vi "LBCB Initialization & Autobalancing.vi"(0 "Selected LBCB":T1, 3 "error in (no error)":errorcluster) -> (8 "Use Previous\nCommand":bool, 10 "error out":errorcluster)   [LabVIEW 2009]
uses:
  lib/Data Access Objects/Metadata/LBCB Number.ctl
  lib/Global Data/Transactions/Dataset Transaction Id.ctl
  lib/Global Data/Transactions/Dataset Source.ctl
  lib/Global Data/Transactions/Dataset Type.ctl
  lib/Apps/Yes No Button.ctl
  lib/Data Access Objects/Metadata/DAO Actions.ctl
panel:
  in  "Autobalance":bool
  in  "Previous Command":bool
  out "Current Displacements":dbl[](array[numeric])
  in  "Previous Command Values":dbl[](array[numeric])
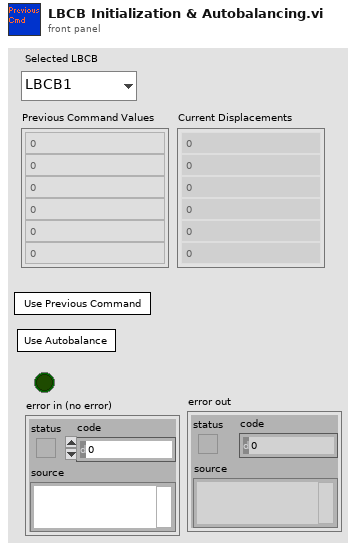
[diagram p1: front panel]
types:
  T1 = typedef "LBCB Number.ctl" = enum16{"LBCB1", "LBCB2"}
  T2 = typedef "Dataset Transaction Id.ctl" = cluster{"Dataset Source":T3, "Dataset Type":T4, "Hold":T5, "Volts":T5, "Tag":string}
  T3 = typedef "Dataset Source.ctl" = enum16{"LBCB 1", "LBCB 2", "Combined", "External Sensors"}
  T4 = typedef "Dataset Type.ctl" = enum16{"LVDT", "Load Cell", "Actuator Command", "Servo Error", "Displacement Command", "Displacement", "Force"}
  T5 = typedef "Yes No Button.ctl" = bool
  T6 = typedef "DAO Actions.ctl" = enum16{"Init", "Get", "Set"}
  T7 = typedef "Actuator Point.ctl" = cluster{"X1":dbl, "X2":dbl, "Y1":dbl, "Z1":dbl, "Z2":dbl, "Z3":dbl}
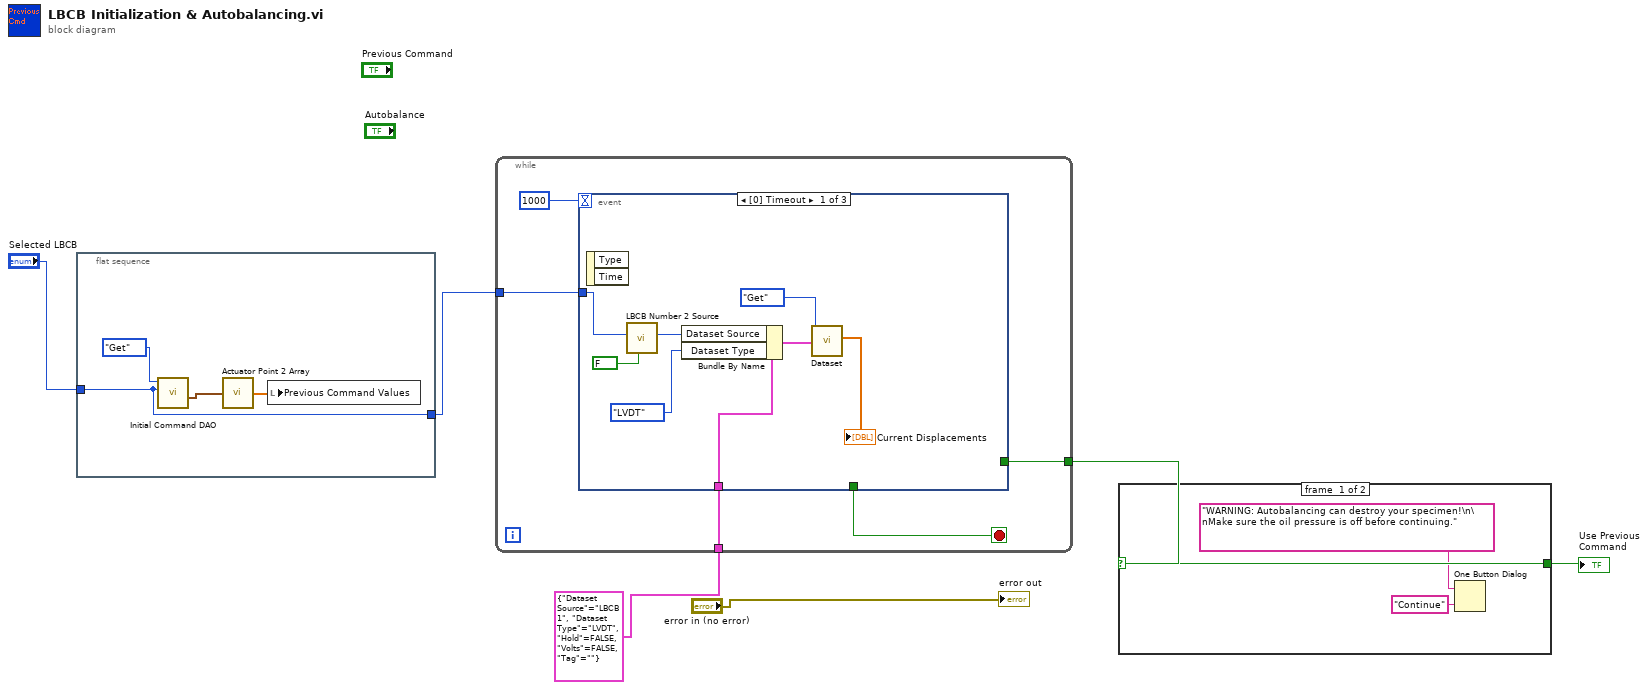
[diagram p0: block diagram]
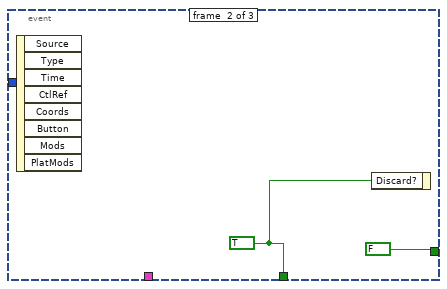
[diagram p3: hidden frame]
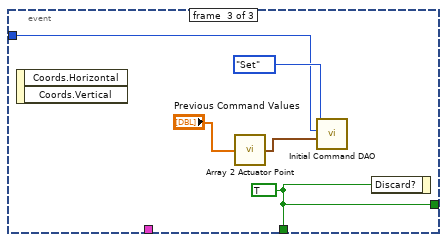
[diagram p4: hidden frame]
diagram:
  n1 = flat-sequence {
    tunnel: "Selected LBCB" -> [w7]
    tunnel: [w7] -> w2
    frame #0 {
      n2 = call "Initial Command DAO.vi"("LBCB Number"=w7, "DAO Actions"=DAO_Actions."Get") -> ("Command Out"=w9:T7)  [unwired: 2 in, 7 out]
      n3 = call "Actuator Point 2 Array.vi"("Actuator Point"=w9) -> ("Array"=w8:dbl[])
      n4 = local write "Previous Command Values"(w8) -> ()
    }
  }
  n5 = while {
    tunnel: [w13] -> w4
    tunnel: w2 -> [w12]
    tunnel: T2 {"Dataset Source"=enum."LBCB 1", "Dataset Type"=enum."LVDT", "Hold"=FALSE, "Volts"=FALSE, "Tag"=""} ("Dataset Trans Id") -> [w11]
    stop <- w14 stop-if-true
    n6 = event shown="[0] Timeout" {
      selector: _ -> [_ _ _]
      dyn-events: _ -> [_ _ _]
      timeout: 1000 -> [_ _ _]
      tunnel: [_ w24 w26] -> w14
      tunnel: [_ FALSE w26] -> w13
      tunnel: w12 -> [w23 _ w27]
      tunnel: w11 -> [w22 _ _]
      event #0 {
        n7 = event-data() -> ()  [unwired: 3 out]
        n8 = call "LBCB Number 2 Source.vi"("Combined"=FALSE, "LBCB Number"=w23) -> ("Dataset Source"=w21:T3)  [unwired: 9 in]
        n9 = Bundle By Name(cluster=w22, "Dataset Source"=w21, "Dataset Type"=Dataset_Type."LVDT") -> (w19:T2)
        n10 = call "Dataset.vi"("Dataset Trans Id"=w19, "DAO Actions"=DAO_Actions."Get") -> ("Data Out"=→"Current Displacements":dbl[])  [unwired: 8 in, 1 out]
      }
      event #1 {
        w24 = TRUE
        n11 = event-data() -> ()  [unwired: 9 out]
        n12 = event-data("Discard?"=w24) -> ()  [unwired: 1 in, 1 out]
      }
      event #2 {
        w26 = TRUE
        n13 = event-data() -> ()  [unwired: 3 out]
        n14 = call "Array 2 Actuator Point.vi"("Array"="Previous Command Values") -> ("Actuator Point"=w28:T7)
        n15 = call "Initial Command DAO.vi"("Command In"=w28, "LBCB Number"=w27, "DAO Actions"=DAO_Actions."Set") -> ()  [unwired: 1 in, 8 out]
        n16 = event-data("Discard?"=w26) -> ()  [unwired: 1 in, 1 out]
      }
    }
  }
  n17 = case shown="False" w4 {
    selector: w4 -> [w33 w34]
    tunnel: [w33 w34] -> w3
    frame #0 {
      n18 = One Button Dialog(message="WARNING: Autobalancing can destroy your specimen!\n\nMake sure the oil pressure is off before continuing." ("string"), button name ("OK")="Continue") -> ()  [unwired: 1 out]
    }
    frame #1 {
    }
  }
  "Use Previous\nCommand" <- w3
  "error out" <- "error in (no error)"
